vi "UpConvert AssertEventData.vi"(10 "Assert Event Data":T1={"Name"="", "Passed"=FALSE, "Call Chain"=[], "Test Error"={"status"=FALSE, "code"=0, "source"=""}, "Time Stamp"=timestamp(0 s since 1904-01-01), "Unique Assert ID"="", "Test ID"="", "Execution time (s)"=-1.0, "Verbose Explanation"=""}) -> (2 "Assert Event Data (Extended)":T2={"name"="", "Passed"=FALSE, "call-chain"=[], "Test Error"={"status"=FALSE, "code"=0, "source"=""}, "timestamp"=timestamp(0 s since 1904-01-01), "assert-id"="", "test-id"="", "time"=-1.0, "message"="", "properties"=variant, "measurements"=variant, "user-defined"=variant})   [LabVIEW 2013, in "Caraya.lvlib" / "Test Result.lvclass"]
uses:
  Test Result.lvclass
  Assert Event Data (Extended).ctl
  Assert Event Data.ctl
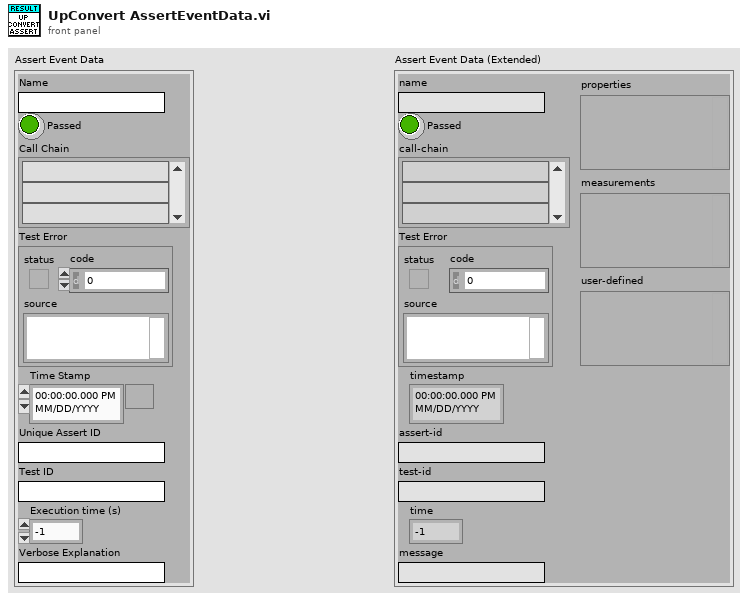
[diagram p1: front panel]
types:
  T1 = typedef "Caraya.lvlib/Test Result.lvclass/Assert Event Data.ctl" = cluster{"Name":string, "Passed":bool, "Call Chain":string[], "Test Error":errorcluster, "Time Stamp":timestamp, "Unique Assert ID":string, "Test ID":string, "Execution time (s)":dbl, "Verbose Explanation":string}
  T2 = typedef "Caraya.lvlib/Test Result.lvclass/Assert Event Data (Extended).ctl" = cluster{"name":string, "Passed":bool, "call-chain":string[], "Test Error":errorcluster, "timestamp":timestamp, "assert-id":string, "test-id":string, "time":dbl, "message":string, "properties":variant, "measurements":variant, "user-defined":variant}
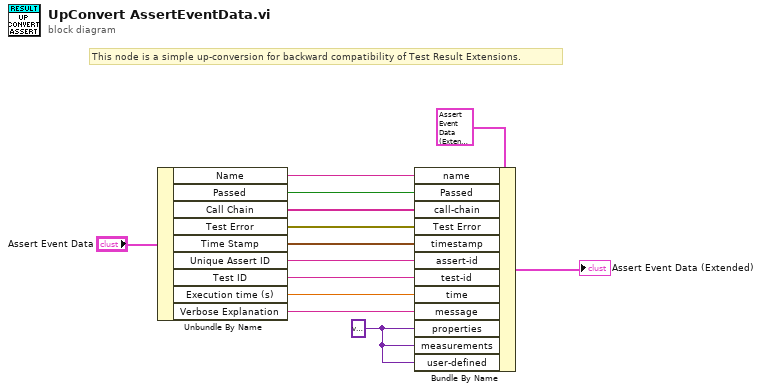
[diagram p0: block diagram]
diagram:
  w2 = variant ("properties")
  # "This node is a simple up-conversion for backward compatibility of Test Result Extensions."
  n1 = Unbundle By Name("Assert Event Data") -> ("Name"=w13:string, "Passed"=w12:bool, "Call Chain"=w11:string[], "Test Error"=w10:errorcluster, "Time Stamp"=w9:timestamp, "Unique Assert ID"=w8:string, "Test ID"=w7:string, "Execution time (s)"=w6:dbl, "Verbose Explanation"=w5:string)
  n2 = Bundle By Name(cluster=T2 {"name"="", "Passed"=FALSE, "call-chain"=[], "Test Error"={"status"=FALSE, "code"=0, "source"=""}, "timestamp"=timestamp(0 s since 1904-01-01), "assert-id"="", "test-id"="", "time"=-1.0, "message"="", "properties"=variant, "measurements"=variant, "user-defined"=variant} ("Assert Event Data (Extended)"), "name"=w13, "Passed"=w12, "call-chain"=w11, "Test Error"=w10, "timestamp"=w9, "assert-id"=w8, "test-id"=w7, "time"=w6, "message"=w5, "properties"=w2, "measurements"=w2, "user-defined"=w2) -> (→"Assert Event Data (Extended)":T2)
